vi "Labspec PutValue.vi"(6 "pValue":variant, 8 "error in":errorcluster, 9 "Name":T1, 10 "DataID":i32, 11 "Automation Refnum In":refnum<k7>) -> (0 "error out":errorcluster, 2 "Succeded?":bool, 3 "Automation Refnum Out":refnum<k7>)   [LabVIEW 2014]
uses:
  PutValue Name.ctl
panel:
  out "PutValue":i32
  # "LICENSED MATERIALS – PROPERTY OF IBM\nCopyright IBM Corp. 2016,\nALL RIGHTS RESERVED"
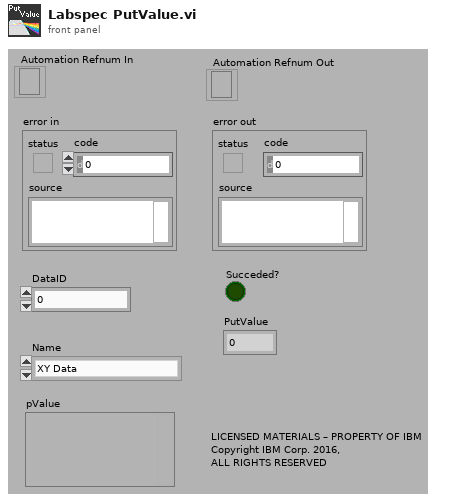
[diagram p1: front panel]
types:
  T1 = typedef "PutValue Name.ctl" = enum16{"XY Data", "Data", "MapPoint:SpectrumIndex", "Axis Labels", "Axis Units", "Axis", "Axis Limits", "Frequency Unit", "Intensity Unit", "Cursor Type", "Pointer Limits", "Active Cursors", "Special Script Type", "CCD Shutter", "Laser", "SWIFT", "Labspec Exposure Time", "Labspec Accumulation", "Active Frame"}
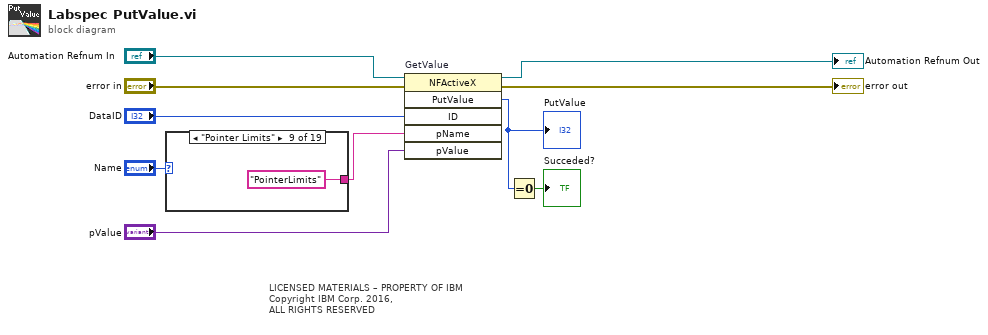
[diagram p0: block diagram]
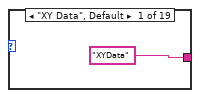
[diagram p2: hidden frame]
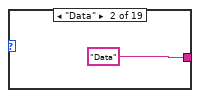
[diagram p3: hidden frame]
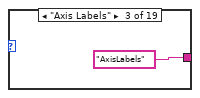
[diagram p4: hidden frame]
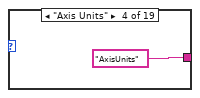
[diagram p5: hidden frame]
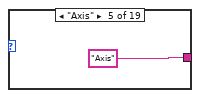
[diagram p6: hidden frame]
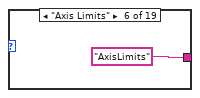
[diagram p7: hidden frame]
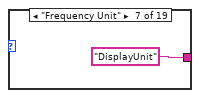
[diagram p8: hidden frame]
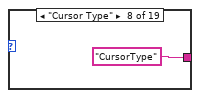
[diagram p9: hidden frame]
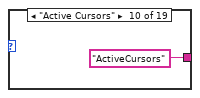
[diagram p10: hidden frame]
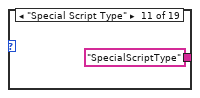
[diagram p11: hidden frame]
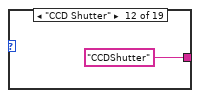
[diagram p12: hidden frame]
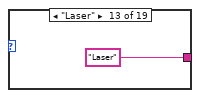
[diagram p13: hidden frame]
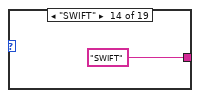
[diagram p14: hidden frame]
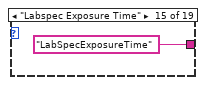
[diagram p15: hidden frame]
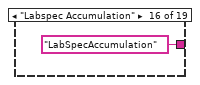
[diagram p16: hidden frame]
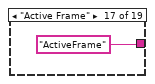
[diagram p17: hidden frame]
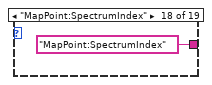
[diagram p18: hidden frame]
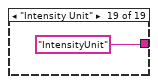
[diagram p19: hidden frame]
diagram:
  # "LICENSED MATERIALS – PROPERTY OF IBM\nCopyright IBM Corp. 2016,\nALL RIGHTS RESERVED"
  n1 = case shown="\"Pointer Limits\"" "Name" {
    tunnel: ["XYData" "Data" "AxisLabels" "AxisUnits" "Axis" "AxisLimits" "DisplayUnit" "CursorType" "PointerLimits" "ActiveCursors" "SpecialScriptType" "CCDShutter" "Laser" "SWIFT" "LabSpecExposureTime" "LabSpecAccumulation" "ActiveFrame" "MapPoint:SpectrumIndex" "IntensityUnit"] -> w4
    frame "XY Data", Default {
    }
    frame "Data" {
    }
    frame "Axis Labels" {
    }
    frame "Axis Units" {
    }
    frame "Axis" {
    }
    frame "Axis Limits" {
    }
    frame "Frequency Unit" {
    }
    frame "Cursor Type" {
    }
    frame "Pointer Limits" {
    }
    frame "Active Cursors" {
    }
    frame "Special Script Type" {
    }
    frame "CCD Shutter" {
    }
    frame "Laser" {
    }
    frame "SWIFT" {
    }
    frame "Labspec Exposure Time" {
    }
    frame "Labspec Accumulation" {
    }
    frame "Active Frame" {
    }
    frame "MapPoint:SpectrumIndex" {
    }
    frame "Intensity Unit" {
    }
  }
  n2 = invoke on="GetValue" class="NFActiveX" method="PutValue"(reference="Automation Refnum In", error in="error in", "ID"="DataID", "pName"=w4, "pValue"="pValue") -> (reference out=→"Automation Refnum Out":refnum<k7>, error out=→"error out":errorcluster, "PutValue"=w3:i32)  [unwired: 1 in, 3 out]
  "PutValue" <- w3
  n3 = Equal To 0?(x=w3) -> (x = 0?=→"Succeded?":bool)
